vi "read.vi"(8 "error in (no error)":errorcluster, 11 "TCPConnection In":refnum<class "TCPConnection.lvclass">) -> (0 "error out":errorcluster, 2 "message":string, 3 "TCPConnection Out":refnum<class "TCPConnection.lvclass">)   [LabVIEW 2023, in "AbstractFactory.lvlib" / "TCPConnection.lvclass"]
uses:
  TCPConnection.lvclass
  TCPConnection.lvclass/TCPConnection.ctl
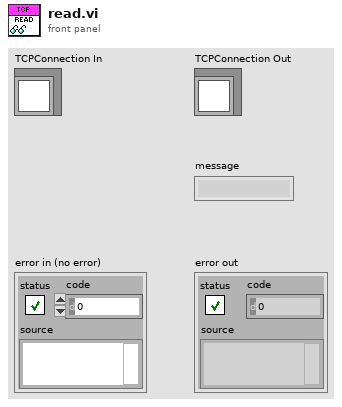
[diagram p1: front panel]
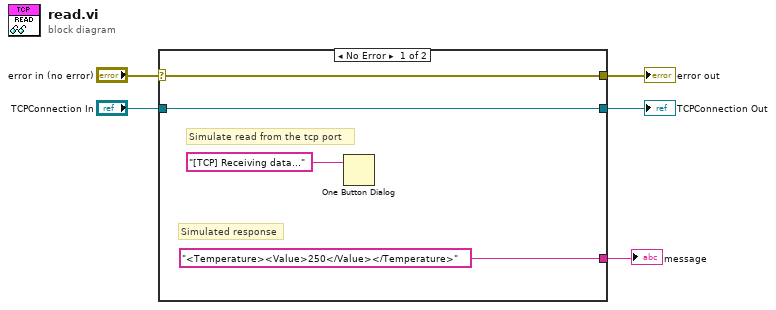
[diagram p0: block diagram]
diagram:
  n1 = case shown="No Error" "error in (no error)" {
    selector: "error in (no error)" -> [w8 w11]
    tunnel: [w8 w11] -> w4
    tunnel: [w9 w10] -> w3
    tunnel: "TCPConnection In" -> [w9 w10]
    tunnel: ["<Temperature><Value>250</Value></Temperature>" ("message") _] -> w1
    frame No Error {
      # "Simulated response"
      # "Simulate read from the tcp port"
      n2 = One Button Dialog(message="[TCP] Receiving data..." ("format string")) -> ()  [unwired: 1 in, 1 out]
    }
    frame Error {
    }
  }
  "error out" <- w4
  "TCPConnection Out" <- w3
  "message" <- w1
